vi "界面UI.vi"() -> ()   [LabVIEW 2016, in "德润DR803M超标留样.lvlib"]
uses:
  <vilib>/Utility/miscctls.llb/LVPointTypeDef.ctl
  <vilib>/Utility/config.llb/NI_LVConfig.lvlib
panel:
  in  "超标浓度配置":bool
  out "超标留样等待时间/s":dbl
  in  "流程停止":bool
  in  "流程启动":bool
  out "流程中":bool
  out "超标留样运行状态":T1(xcontrol)
  in  "外控留样设置":bool
  in  "外控留样读取":bool
  in  "串口重开":bool
  in  "读取选择":string(combo)
  in  "超标留样设置":bool
  in  "超标留样读取":bool
  in  "VISA resource name":refnum<visa-resource-name>="COM10" caption="VISA资源名称"
  in  "写入缓冲区":string
  in  "采样模式":enum16{"定时留样", "时间等比", "同步留样", "外控留样", "超标留样"}(ring)
  in  "采样启动":bool
  in  "切换停止":bool
  in  "切换运行":bool
  in  "时间校准":bool
  out "仪器状态":T1 {"仪器时间" format="%<%Y/%m/%d %H:%M:%S>T"; "门状态" items=["关闭", "打开"]; "采样模式" items=["定时留样"=1, "时间等比"=2, "同步留样"=3, "外控留样"=4, "超标留样"=5]; "工作进程" items=["停止中"=0, "启动延时"=1, "外置泵延时"=2, "管路润洗"=3, "管存"=4, "留样"=5, "出水管路排空"=6, "采水管路排空"=7, "待机"=13]; "工作状态" items=["停止", "运行", "系统初始化"]}
  out "读取缓冲区":string
  out "source":string
  out "通讯":bool
  # "德润超标留样803M"
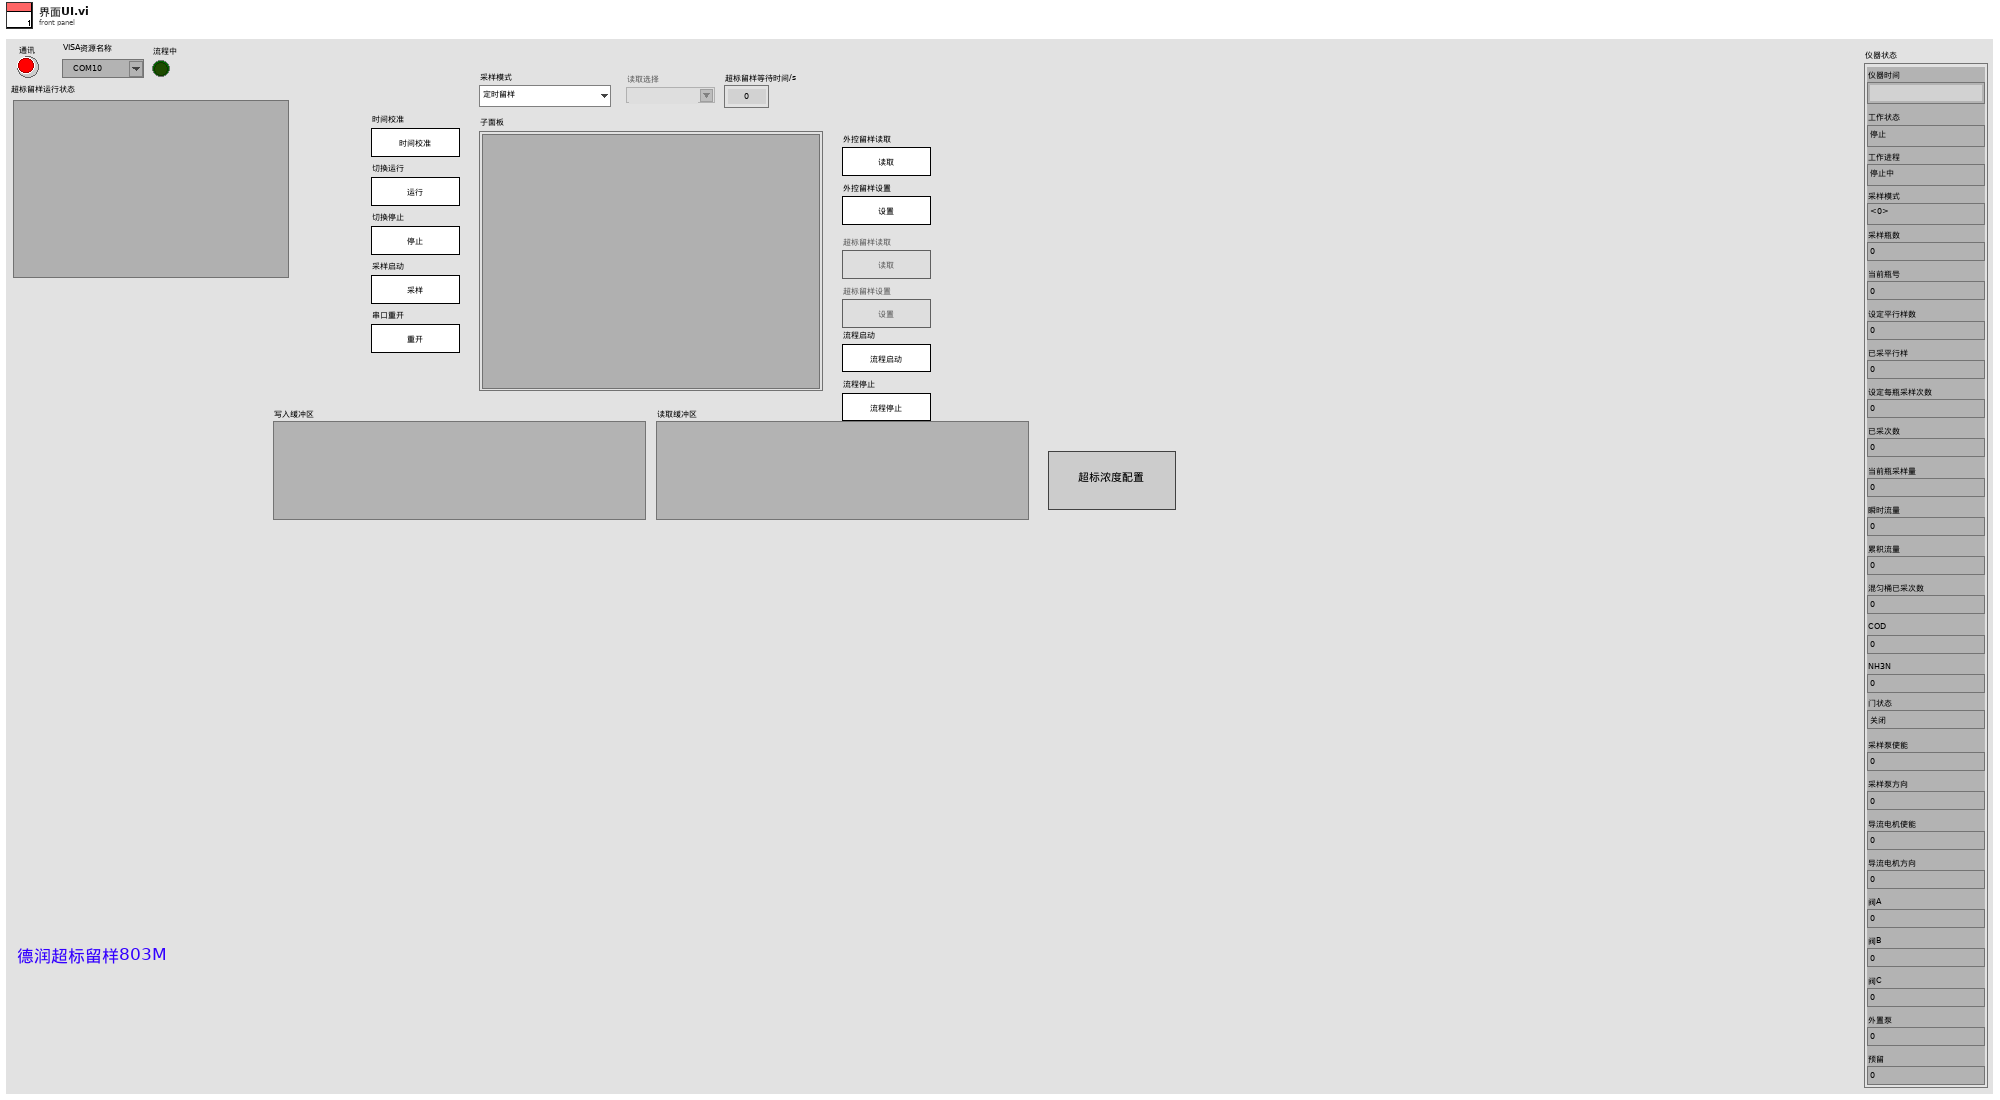
[diagram p1: front panel]
types:
  T1 = cluster{"仪器时间":timestamp, "工作状态":u16, "工作进程":u16, "采样模式":u16, "采样瓶数":dbl, "当前瓶号":dbl, "设定平行样数":dbl, "已采平行样":dbl, "设定每瓶采样次数":dbl, "已采次数":dbl, "当前瓶采样量":dbl, "瞬时流量":dbl, "累积流量":dbl, "混匀桶已采次数":dbl, "COD":dbl, "NH3N":dbl, "门状态":u16, "采样泵使能":dbl, "采样泵方向":dbl, "导流电机使能":dbl, "导流电机方向":dbl, "阀A":dbl, "阀B":dbl, "阀C":dbl, "外置泵":dbl, "预留":dbl}
  T2 = cluster{"STEP":enum16{"open", "read", "write", "close"}, "写入缓冲区":string}
  T3 = typedef "LVPointTypeDef.ctl" = cluster{"Horizontal":i16, "Vertical":i16}
  T4 = typedef "NI_LVConfig.lvlib/Config Data RefNum.ctl" = refnum<k1>
  T5 = enum32{"Bad", "Idle", "Run top level", "Running"}
  T6 = cluster{"当前瓶号：":dbl, "平行样：":dbl, "留样瓶数：":dbl, "每瓶次数：":dbl, "每次留样：":dbl}
  T7 = cluster{"当前瓶号：":dbl, "平行样：":dbl, "留样瓶数：":dbl, "每瓶次数：":dbl, "每次留样：":dbl, "时间间隔：":dbl, "COD联机：":u16, "氨氮联机：":u16, "4mA浓度：":dbl, "20mA浓度：":dbl, "超标浓度：":dbl, "4mA浓度：":dbl, "20mA浓度:":dbl, "超标浓度：":dbl}
  T8 = cluster{"[0]":dbl, "[1]":dbl, "[2]":dbl, "[3]":dbl, "[4]":dbl}
  T9 = cluster{"确定":bool, "氨氮超标浓度":dbl, "总磷超标浓度":dbl, "总氮超标浓度":dbl, "CODMn超标浓度":dbl, "CODCr超标浓度":dbl}
  T10 = enum8{"Enabled", "Disabled", "Disabled and Grayed Out"}
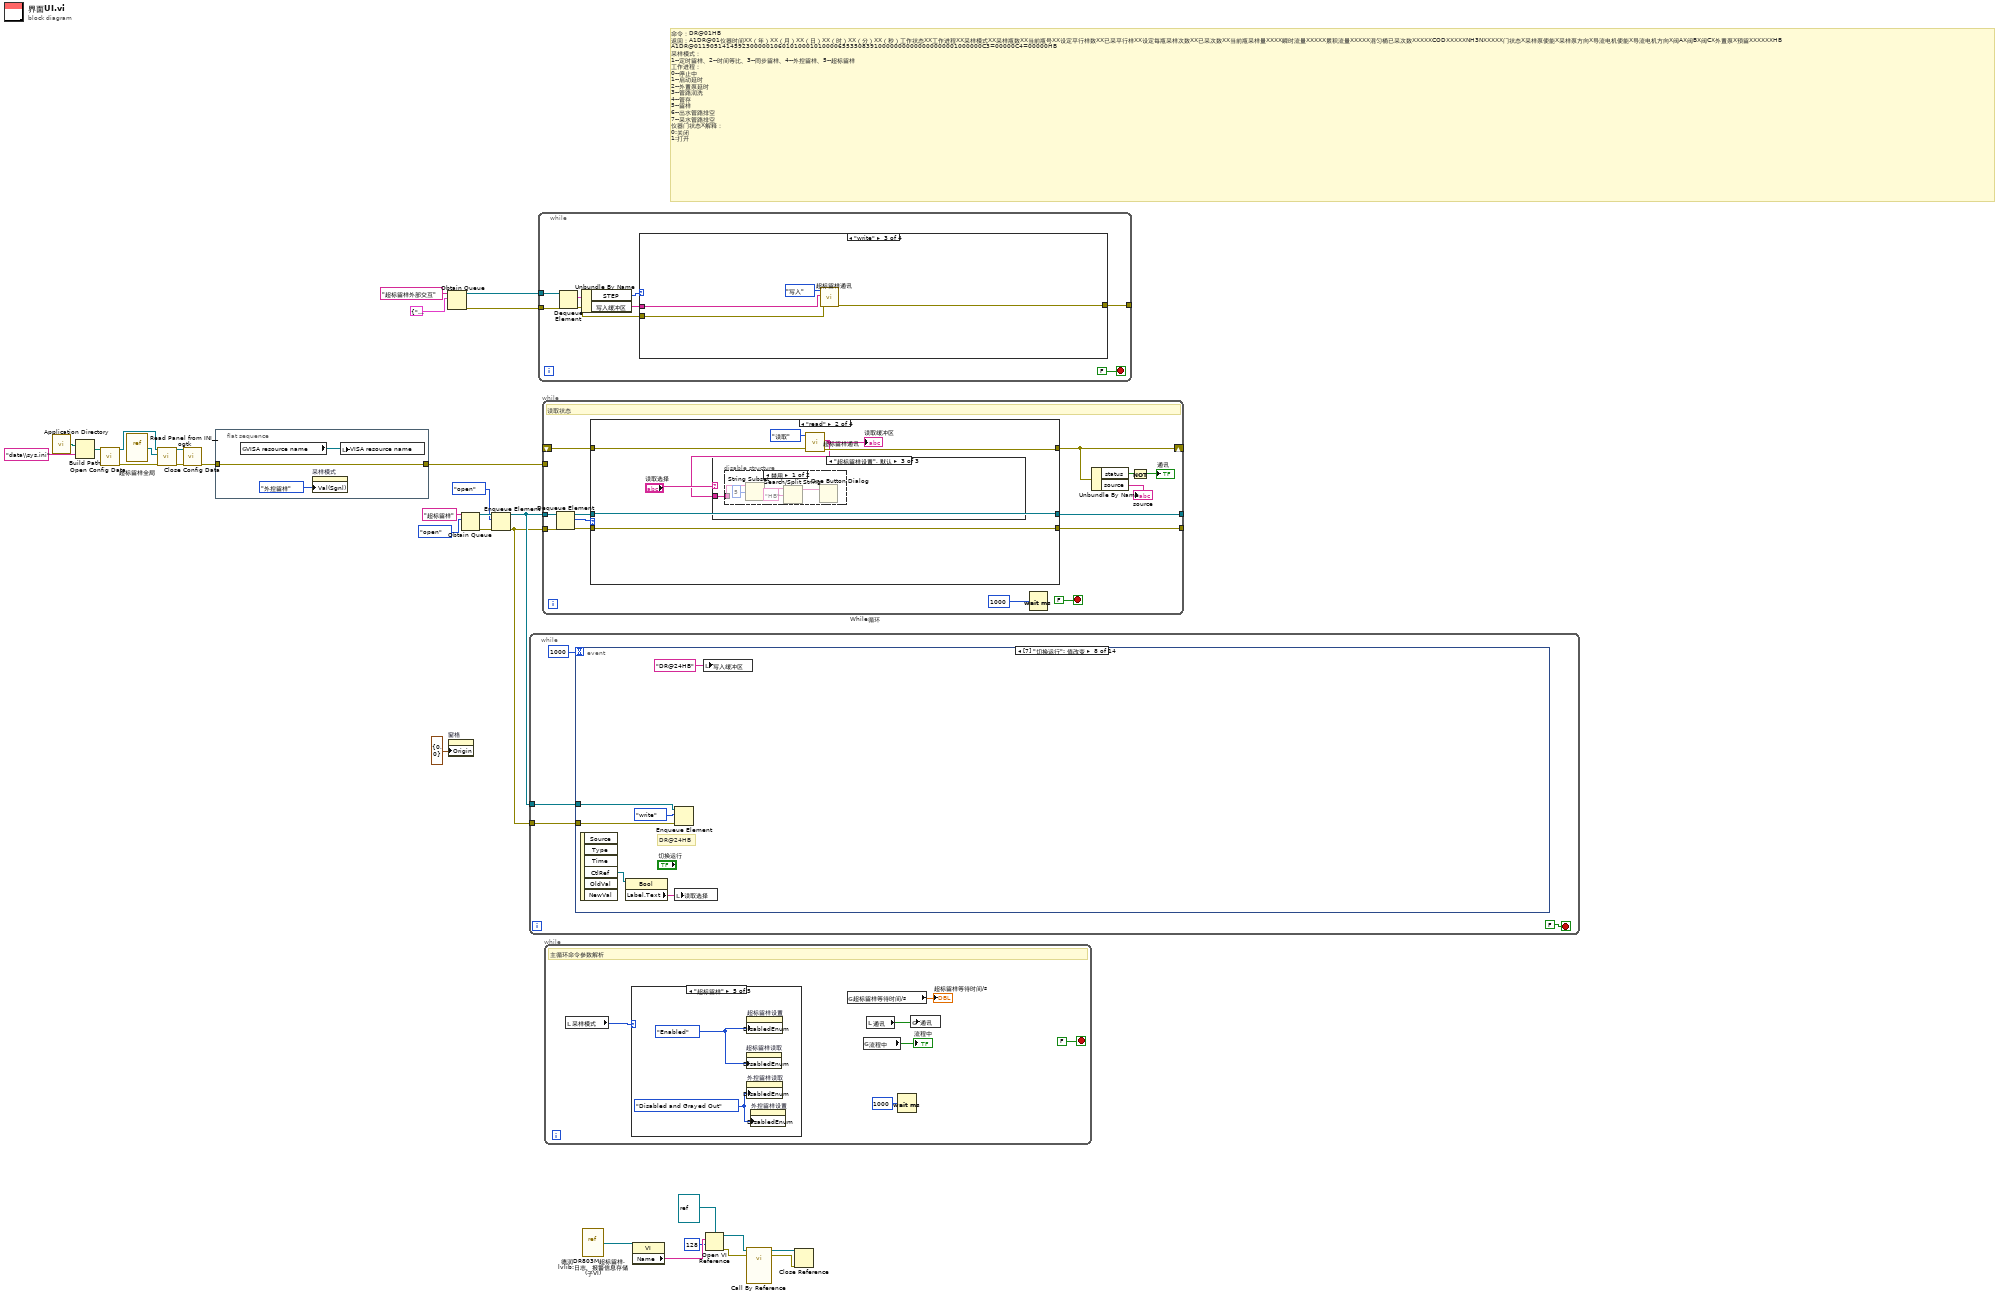
[diagram p0: block diagram]
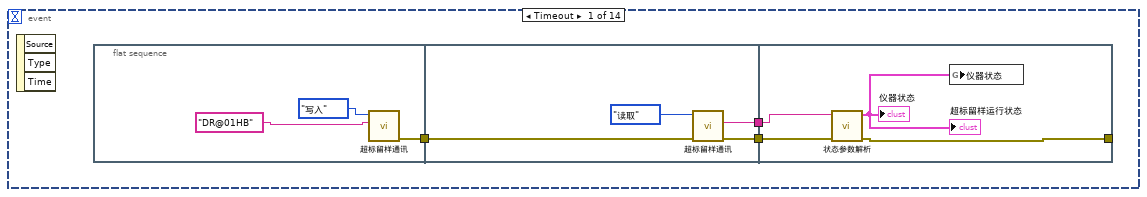
[diagram p5: hidden frame]
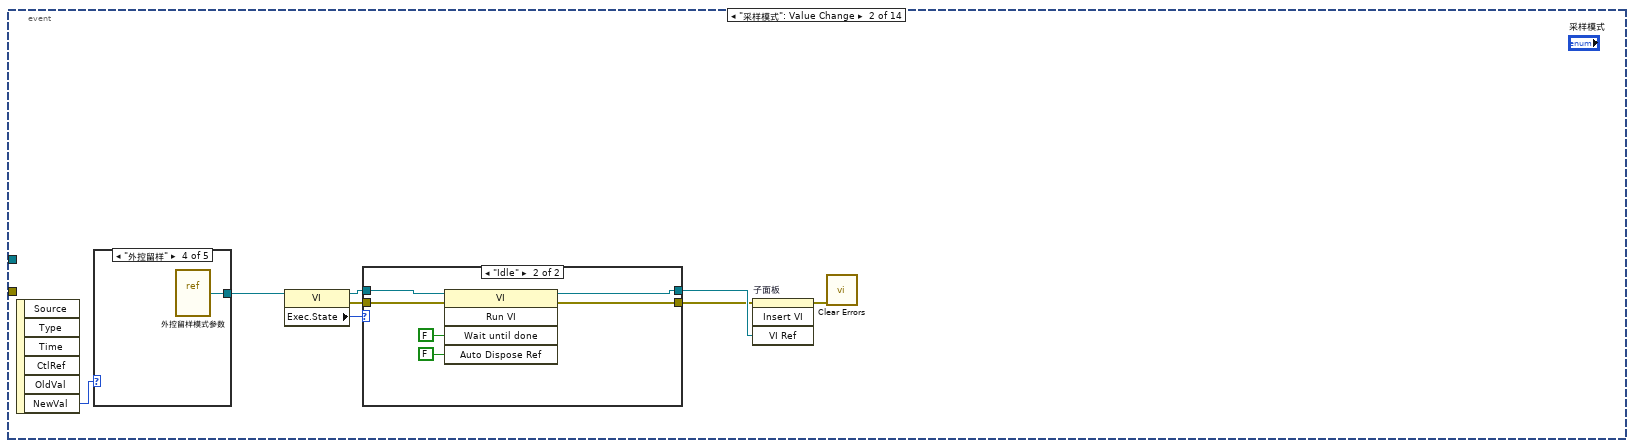
[diagram p6: hidden frame]
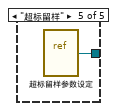
[diagram p11: hidden frame]
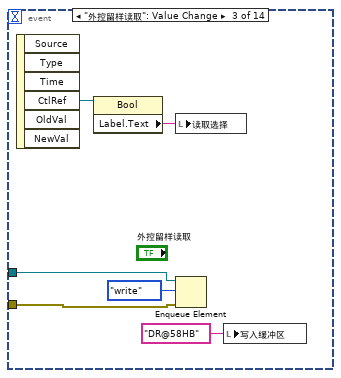
[diagram p12: hidden frame]
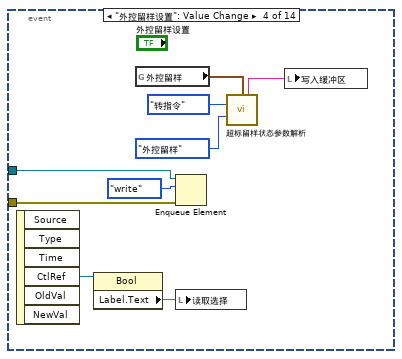
[diagram p13: hidden frame]
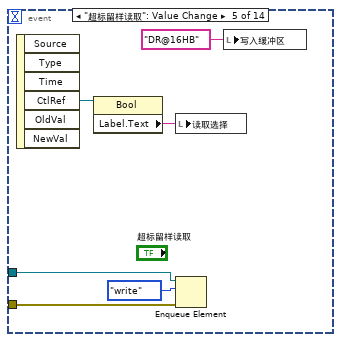
[diagram p14: hidden frame]
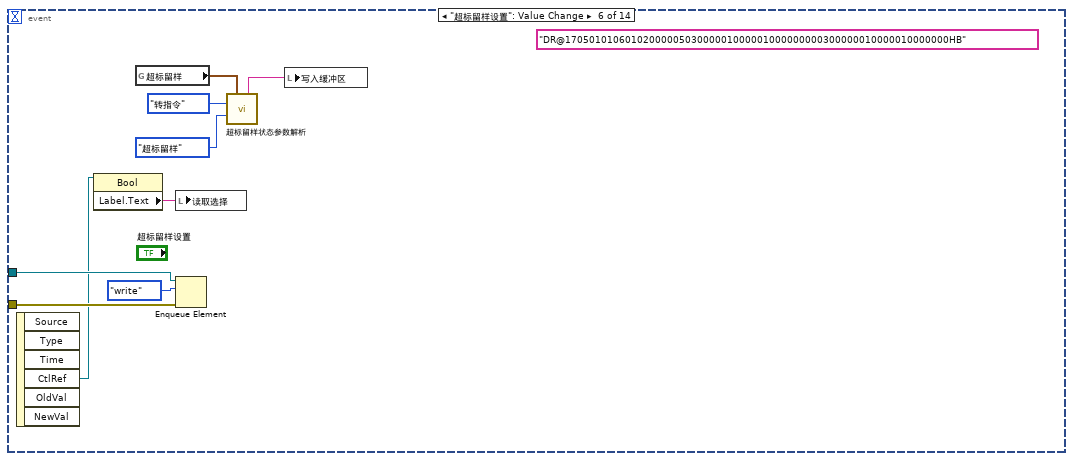
[diagram p15: hidden frame]
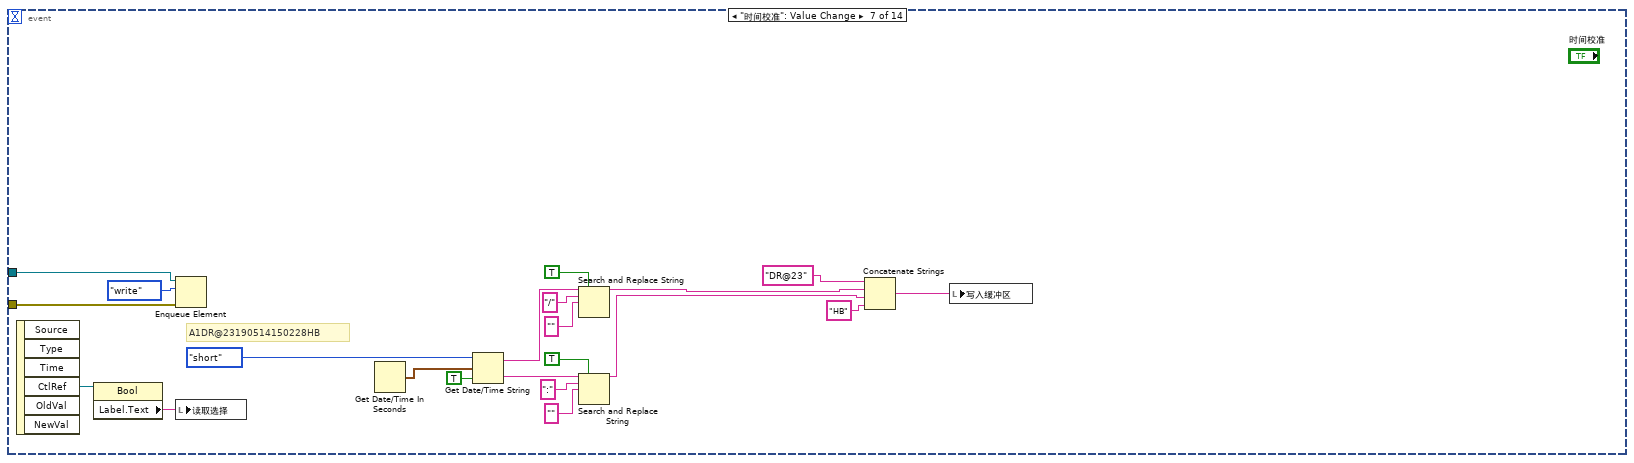
[diagram p16: hidden frame]
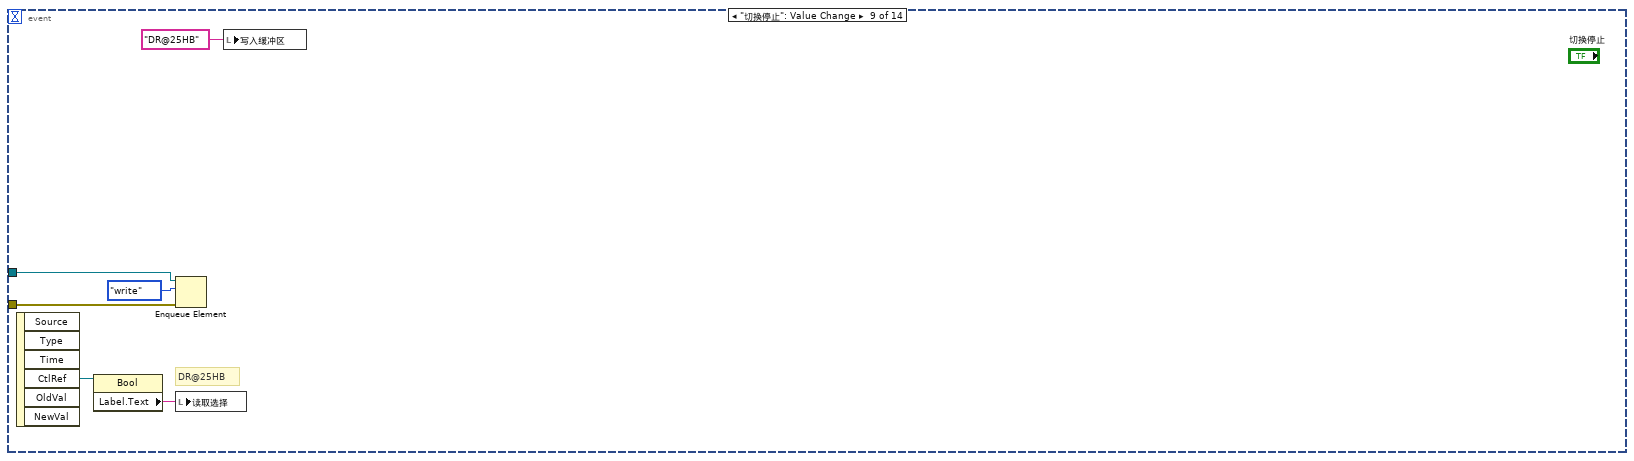
[diagram p17: hidden frame]
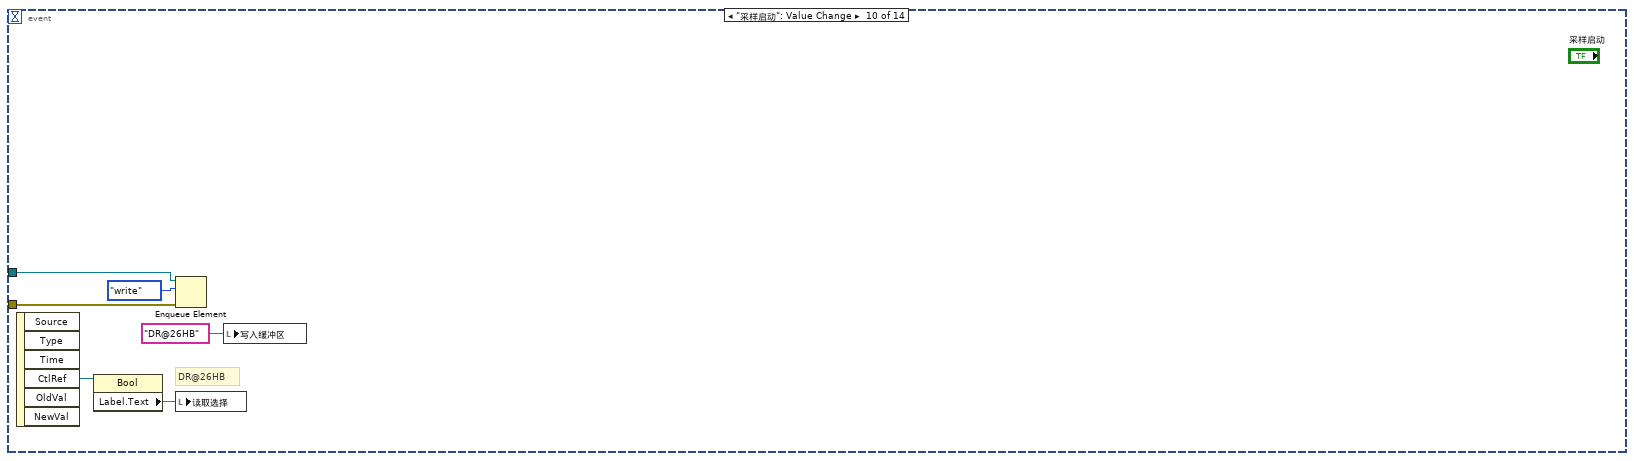
[diagram p18: hidden frame]
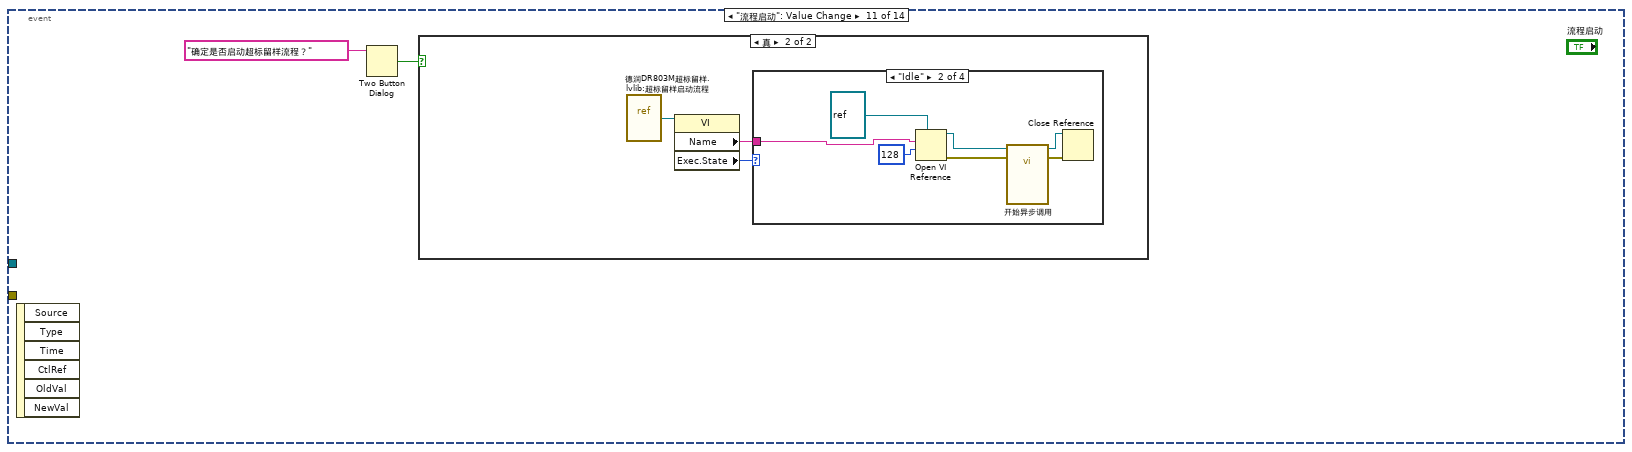
[diagram p19: hidden frame]
diagram:
  # "命令：DR@01HB\n返回：A1DR@01仪器时间XX（年）XX（月）XX（日）XX（时）XX（分）XX（秒）工作状态XX工作进程XX采样模式XX采样瓶数XX当前瓶号XX设定平行样数XX已采平行样XX设定每瓶采样次数XX已采次数XX当前瓶采样量XXXX瞬时流量XXXXX累积流量XXXXX混匀桶已采次数XXXXXCODXXXXXNH3NXXXXX门状态X采样泵使能X采样泵方向X导流电机使能X导流电机方向X阀AX阀BX阀CX外置泵X预留XXXXXXHB\nA1DR@011905141459230000010601010001010000655350839100000000000000000001000000C3=00000C4=00000HB\n采样模式：\n1--定时留样、2--时间等比、3--同步留样、4--外控留样、5--超标留样\n工作进程：\n0--停止中\n1--启动延时\n2--外置泵延时\n3--管路润洗\n4--管存\n5--留样\n6--出水管路排空\n7--采水管路排空\n仪器门状态X解释：\n0:关闭\n1:打开"
  n1 = call <vilib>:"Application Directory.vi"() -> ("Application Directory"=w22:path)
  n2 = Build Path(base path=w22, name or relative path="data\\sys.ini" ("名称或相对路径")) -> (appended path=w20:path)
  n3 = call <vilib>:"Open Config Data.vi"("configuration file path"=w20) -> ("error out"=w16:errorcluster, "refnum"=w19:T4)  [unwired: 8 in, 1 out]
  n4 = vi-ref "超标留样全局.vi"() -> (w18:refnum<vi>)
  n5 = call <userlib>:"Read Panel from INI__ogtk.vi"("error in (no error)"=w16, "VI ref"=w18, "refnum"=w19) -> ("error out"=w15:errorcluster, "refnum out"=w17:T4)  [unwired: 7 in]
  n6 = call <vilib>:"Close Config Data.vi"("error in (no error)"=w15, "refnum"=w17) -> ("error out"=w14:errorcluster)  [unwired: 8 in, 1 out]
  n7 = flat-sequence {
    tunnel: w14 -> [w33]
    tunnel: [w33] -> w13
    frame #0 {
      n8 = global read "超标留样全局.vi" "VISA resource name"() -> (w32:refnum<visa-resource-name>)
      n9 = property on="采样模式" class="Enum (严格)"("Val(Sgnl)"=enum16{"定时留样", "时间等比", "同步留样", "外控留样", "超标留样"}."外控留样" ("采样模式")) -> ()  [unwired: 2 in, 2 out]
      n10 = local write "VISA resource name"(w32) -> ()
    }
  }
  n11 = Obtain Queue(name (unnamed)="超标留样外部交互" ("名称（未命名）"), element data type=T2 {"STEP"=enum."write", "写入缓冲区"="ª\u0006\u0000\u0000P`\u00000»"}) -> (queue out=w11:refnum<queue>, error out=w10:errorcluster)  [unwired: 3 in, 1 out]
  n12 = property on="窗格" class="Pane"("Origin"=T3 {"Horizontal"=0, "Vertical"=0} ("原点")) -> ()  [unwired: 2 in, 2 out]
  n13 = Obtain Queue(name (unnamed)="超标留样" ("名称（未命名）"), element data type=enum16{"open", "read", "write", "close"}."open") -> (queue out=w28:refnum<queue>, error out=w27:errorcluster)  [unwired: 3 in, 1 out]
  n14 = Enqueue Element(queue=w28, element=enum16{"open", "read", "write", "close"}."open", error in (no error)=w27) -> (queue out=w25:refnum<queue>, error out=w24:errorcluster)  [unwired: 1 in, 1 out]
  n15 = while {
    tunnel: w25 -> [w36]
    tunnel: w24 -> [w35]
    stop <- FALSE stop-if-true
    n16 = event shown="[7] \"切换运行\": 值改变" {
      selector: _ -> [_ _ _ _ _ _ _ _ _ _ _ _ _ _]
      dyn-events: _ -> [_ _ _ _ _ _ _ _ _ _ _ _ _ _]
      timeout: 1000 -> [_ _ _ _ _ _ _ _ _ _ _ _ _ _]
      tunnel: w36 -> [_ _ w72 w83 w88 w98 w119 w124 w130 w136 _ w153 w168 _]
      tunnel: w35 -> [_ _ w73 w82 w87 w97 w118 w123 w129 w135 _ w152 w167 _]
      event Timeout {
        n17 = event-data() -> ()  [unwired: 1 in, 3 out]
        n18 = flat-sequence {
          tunnel: [w41] -> w40
          tunnel: w40 -> [w46]
          tunnel: [w45] -> w39
          tunnel: [w44] -> w38
          tunnel: w39 -> [w51]
          tunnel: w38 -> [w50]
          tunnel: [w49] -> _
          frame #0 {
            n19 = call "超标留样通讯.vi"("写入缓冲区"="DR@01HB", "功能输入"=enum16{"打开串口", "写入", "读取", "关闭串口"}."写入") -> ("error out"=w41:errorcluster)  [unwired: 7 in, 2 out]
          }
          frame #1 {
            n20 = call "超标留样通讯.vi"("error in (no error)"=w46, "功能输入"=enum16{"打开串口", "写入", "读取", "关闭串口"}."读取") -> ("error out"=w45:errorcluster, "读取缓冲区"=w44:string)  [unwired: 7 in, 1 out]
          }
          frame #2 {
            n21 = call "状态参数解析.vi"("error in (no error)"=w51, "字符串"=w50) -> ("error out"=w49:errorcluster, "簇"=w48:T1)  [unwired: 8 in]
            "仪器状态" <- w48
            "超标留样运行状态" <- w48
            n22 = global write "超标留样全局.vi" "仪器状态"(w48) -> ()
          }
        }
      }
      event "采样模式": Value Change {
        n23 = event-data() -> ("NewVal"=w59:enum16{"定时留样", "时间等比", "同步留样", "外控留样", "超标留样"})  [unwired: 1 in, 5 out]
        n24 = case shown="\"外控留样\"" w59 {
          tunnel: [_ _ _ w68 w69] -> w58
          frame "定时留样", Default {
          }
          frame "时间等比" {
          }
          frame "同步留样" {
          }
          frame "外控留样" {
            n25 = vi-ref "外控留样模式参数.vi"() -> (w68:refnum<vi>)
          }
          frame "超标留样" {
            n26 = vi-ref "超标留样参数设定.vi"() -> (w69:refnum<vi>)
          }
        }
        n27 = property class="VI"(reference=w58) -> (reference out=w56:refnum<vi>, error out=w54:errorcluster, "Exec.State"=w57:T5)  [unwired: 1 in]
        n28 = case shown="\"Idle\"" w57 {
          tunnel: w56 -> [w61 w67]
          tunnel: [w61 w64] -> w55
          tunnel: w54 -> [w60 w63]
          tunnel: [w60 w62] -> w53
          frame "Bad", Default {
          }
          frame "Idle" {
            n29 = invoke class="VI" method="Run VI"(reference=w67, error in=w63, "Wait until done"=FALSE ("结束前等待"), "Auto Dispose Ref"=FALSE ("自动销毁引用")) -> (reference out=w64:refnum<vi>, error out=w62:errorcluster)  [unwired: 1 in, 3 out]
          }
        }
        n30 = invoke on="子面板" class="SubPnl" method="Insert VI"(error in=w53, "VI Ref"=w55) -> (error out=w52:errorcluster)  [unwired: 2 in, 3 out]
        n31 = call <vilib>:"Clear Errors.vi"("error in (no error)"=w52) -> ()  [unwired: 5 in, 2 out]
      }
      event "外控留样读取": Value Change {
        n32 = event-data() -> ("CtlRef"=w71:refnum<vi>)  [unwired: 1 in, 5 out]
        n33 = property class="Bool"(reference=w71) -> ("Label.Text"=w70:string)  [unwired: 1 in, 2 out]
        n34 = local write "读取选择"(w70) -> ()
        n35 = Enqueue Element(queue=w72, element=enum16{"open", "read", "write", "close"}."write" ("元素"), error in (no error)=w73) -> ()  [unwired: 1 in, 3 out]
        n36 = local write "写入缓冲区"("DR@58HB") -> ()
      }
      event "外控留样设置": Value Change {
        n37 = event-data() -> ("CtlRef"=w77:refnum<vi>)  [unwired: 1 in, 5 out]
        n38 = property class="Bool"(reference=w77) -> ("Label.Text"=w76:string)  [unwired: 1 in, 2 out]
        n39 = global read "超标留样全局.vi" "外控留样"() -> (w78:T6)
        n40 = Enqueue Element(queue=w83, element=enum16{"open", "read", "write", "close"}."write" ("元素"), error in (no error)=w82) -> ()  [unwired: 1 in, 3 out]
        n41 = local write "读取选择"(w76) -> ()
        n42 = call "超标留样状态参数解析.vi"("外控留样"=w78, "解析/转指令"=enum16{"解析", "转指令"}."转指令", "模式选择"=enum16{"外控留样", "超标留样"}."外控留样") -> ("输出字符串"=w79:string)  [unwired: 11 in, 1 out]
        n43 = local write "写入缓冲区"(w79) -> ()
      }
      event "超标留样读取": Value Change {
        n44 = event-data() -> ("CtlRef"=w86:refnum<vi>)  [unwired: 1 in, 5 out]
        n45 = property class="Bool"(reference=w86) -> ("Label.Text"=w85:string)  [unwired: 1 in, 2 out]
        n46 = local write "读取选择"(w85) -> ()
        n47 = Enqueue Element(queue=w88, element=enum16{"open", "read", "write", "close"}."write" ("元素"), error in (no error)=w87) -> ()  [unwired: 1 in, 3 out]
        n48 = local write "写入缓冲区"("DR@16HB") -> ()
      }
      event "超标留样设置": Value Change {
        (unwired) "DR@1705010106010200000503000001000001000000000300000010000010000000HB"
        n49 = event-data() -> ("CtlRef"=w92:refnum<vi>)  [unwired: 1 in, 5 out]
        n50 = property class="Bool"(reference=w92) -> ("Label.Text"=w91:string)  [unwired: 1 in, 2 out]
        n51 = global read "超标留样全局.vi" "超标留样"() -> (w96:T7)
        n52 = local write "读取选择"(w91) -> ()
        n53 = Enqueue Element(queue=w98, element=enum16{"open", "read", "write", "close"}."write" ("元素"), error in (no error)=w97) -> ()  [unwired: 1 in, 3 out]
        n54 = call "超标留样状态参数解析.vi"("超标留样"=w96, "解析/转指令"=enum16{"解析", "转指令"}."转指令", "模式选择"=enum16{"外控留样", "超标留样"}."超标留样") -> ("输出字符串"=w93:string)  [unwired: 11 in, 1 out]
        n55 = local write "写入缓冲区"(w93) -> ()
      }
      event "时间校准": Value Change {
        # "A1DR@23190514150228HB"
        n56 = event-data() -> ("CtlRef"=w101:refnum<vi>)  [unwired: 1 in, 5 out]
        n57 = property class="Bool"(reference=w101) -> ("Label.Text"=w100:string)  [unwired: 1 in, 2 out]
        n58 = Enqueue Element(queue=w119, element=enum16{"open", "read", "write", "close"}."write" ("元素"), error in (no error)=w118) -> ()  [unwired: 1 in, 3 out]
        n59 = local write "读取选择"(w100) -> ()
        n60 = Get Date/Time In Seconds() -> (seconds since 1Jan1904=w114:timestamp)
        n61 = Get Date/Time String(date format (0)=enum16{"short", "long", "abbreviated"}."short" ("日期格式(0)"), seconds (now)=w114, want seconds? (F)=TRUE ("需要秒？(F)")) -> (date string=w113:string, time string=w106:string)
        n62 = Search and Replace String(replace all?=TRUE ("替换全部？(F)"), input string=w113, search string="/" ("搜索字符串"), replace string="" ("替换字符串(\"\")")) -> (result string=w105:string)  [unwired: 4 in, 3 out]
        n63 = Search and Replace String(replace all?=TRUE ("替换全部？(F)"), input string=w106, search string=":" ("搜索字符串"), replace string="" ("替换字符串(\"\")")) -> (result string=w104:string)  [unwired: 4 in, 3 out]
        n64 = Concatenate Strings("DR@23" ("写入缓冲区"), w105, w104, "HB" ("写入缓冲区")) -> (w102:string)
        n65 = local write "写入缓冲区"(w102) -> ()
      }
      event "切换运行": Value Change {
        # "DR@24HB"
        n66 = event-data() -> ("CtlRef"=w122:refnum<vi>)  [unwired: 1 in, 5 out]
        n67 = property class="Bool"(reference=w122) -> ("Label.Text"=w121:string)  [unwired: 1 in, 2 out]
        n68 = Enqueue Element(queue=w124, element=enum16{"open", "read", "write", "close"}."write" ("元素"), error in (no error)=w123) -> ()  [unwired: 1 in, 3 out]
        n69 = local write "读取选择"(w121) -> ()
        n70 = local write "写入缓冲区"("DR@24HB") -> ()
      }
      event "切换停止": Value Change {
        # "DR@25HB"
        n71 = event-data() -> ("CtlRef"=w128:refnum<vi>)  [unwired: 1 in, 5 out]
        n72 = property class="Bool"(reference=w128) -> ("Label.Text"=w127:string)  [unwired: 1 in, 2 out]
        n73 = Enqueue Element(queue=w130, element=enum16{"open", "read", "write", "close"}."write" ("元素"), error in (no error)=w129) -> ()  [unwired: 1 in, 3 out]
        n74 = local write "读取选择"(w127) -> ()
        n75 = local write "写入缓冲区"("DR@25HB" ("写入缓冲区")) -> ()
      }
      event "采样启动": Value Change {
        # "DR@26HB"
        n76 = event-data() -> ("CtlRef"=w134:refnum<vi>)  [unwired: 1 in, 5 out]
        n77 = property class="Bool"(reference=w134) -> ("Label.Text"=w133:string)  [unwired: 1 in, 2 out]
        n78 = Enqueue Element(queue=w136, element=enum16{"open", "read", "write", "close"}."write" ("元素"), error in (no error)=w135) -> ()  [unwired: 1 in, 3 out]
        n79 = local write "读取选择"(w133) -> ()
        n80 = local write "写入缓冲区"("DR@26HB") -> ()
      }
      event "流程启动": Value Change {
        n81 = event-data() -> ()  [unwired: 1 in, 6 out]
        n82 = Two Button Dialog(message="确定是否启动超标留样流程？" ("消息")) -> (T button?=w139:bool)  [unwired: 2 in]
        n83 = case shown="真" w139 {
          frame False {
          }
          frame True {
            n84 = vi-ref "德润DR803M超标留样.lvlib:超标留样启动流程.vi"() -> (w141:refnum<vi>)
            n85 = property class="VI"(reference=w141) -> ("Name"=w142:string, "Exec.State"=w143:T5)  [unwired: 1 in, 2 out]
            n86 = case shown="\"Idle\"" w143 {
              tunnel: w142 -> [_ w146 _ _]
              frame "Bad", Default {
              }
              frame "Idle" {
                n87 = Open VI Reference(type specifier VI Refnum (for type only)=refnum<vi> refnum ("类型说明符VI引用句柄（仅用于类型）"), vi path=w146, options=128 ("选项")) -> (vi reference=w150:refnum<vi>, error out=w145:errorcluster)  [unwired: 3 in]
                n88 = call-by-ref "开始异步调用"(reference=w150, error in=w145) -> (reference out=w149:refnum<vi>, error out=w144:errorcluster)  [unwired: 12 in]
                n89 = Close Reference(reference=w149, error in (no error)=w144) -> ()  [unwired: 1 out]
              }
              frame "Run top level" {
              }
              frame "Running" {
                n90 = One Button Dialog(message="流程已启动，无需重复启动！" ("消息")) -> ()  [unwired: 1 in, 1 out]
              }
            }
          }
        }
      }
      event "流程停止": Value Change {
        n91 = event-data() -> ()  [unwired: 1 in, 6 out]
        n92 = Two Button Dialog(message="确定是否停止超标留样流程并排空当前瓶？" ("消息")) -> (T button?=w154:bool)  [unwired: 2 in]
        n93 = case shown="真" w154 {
          tunnel: w153 -> [_ w158]
          tunnel: w152 -> [_ w157]
          frame False {
          }
          frame True {
            n94 = Enqueue Element(queue=w158, element=enum16{"open", "read", "write", "close"}."write" ("元素"), error in (no error)=w157) -> ()  [unwired: 1 in, 3 out]
            n95 = local write "写入缓冲区"("DR@25HB" ("写入缓冲区")) -> ()
            n96 = Obtain Notifier(name (unnamed)="超标留样流程" ("名称（未命名）"), notification data type=FALSE ("采样完成")) -> (notifier out=w164:refnum<notifier>, error out=w163:errorcluster)  [unwired: 2 in, 1 out]
            n97 = Send Notification(notification=TRUE ("通知"), notifier=w164, error in (no error)=w163) -> (notifier out=w161:refnum<notifier>, error out=w160:errorcluster)
            n98 = Release Notifier(notifier=w161, error in (no error)=w160) -> ()  [unwired: 1 in, 3 out]
          }
        }
      }
      event "串口重开": Value Change {
        n99 = event-data() -> ()  [unwired: 1 in, 6 out]
        n100 = flat-sequence {
          frame #0 {
            n101 = local read "VISA resource name"() -> (w170:refnum<visa-resource-name>)
            n102 = global write "超标留样全局.vi" "VISA resource name"(w170) -> ()
          }
          frame #1 {
            n103 = call <vilib>:"Application Directory.vi"() -> ("Application Directory"=w172:path)
            n104 = Build Path(base path=w172, name or relative path="data\\sys.ini" ("名称或相对路径")) -> (appended path=w173:path)
            n105 = call <vilib>:"Open Config Data.vi"("configuration file path"=w173) -> ("error out"=w177:errorcluster, "refnum"=w174:T4)  [unwired: 8 in, 1 out]
            n106 = vi-ref "超标留样全局.vi"() -> (w175:refnum<vi>)
            n107 = call <userlib>:"Write Panel to INI__ogtk.vi"("error in (no error)"=w177, "VI ref"=w175, "refnum"=w174) -> ("error out"=w178:errorcluster, "refnum out"=w176:T4)  [unwired: 7 in]
            n108 = call <vilib>:"Close Config Data.vi"("error in (no error)"=w178, "refnum"=w176) -> ("error out"=w183:errorcluster, "file path"=w184:path)  [unwired: 8 in]
            n109 = Open/Create/Replace File(file path (use dialog)=w184, error in=w183) -> (refnum out=w180:refnum<file>, error out=w179:errorcluster)  [unwired: 4 in, 1 out]
            n110 = Flush File(refnum=w180, error in=w179) -> (refnum out=w181:refnum<file>, error out=w182:errorcluster)
            n111 = Close File(refnum=w181, error in=w182) -> ()  [unwired: 2 out]
          }
        }
        n112 = Enqueue Element(queue=w168, element=enum16{"open", "read", "write", "close"}."close" ("元素"), error in (no error)=w167) -> ()  [unwired: 1 in, 3 out]
      }
      event "超标浓度配置": Value Change {
        n113 = event-data() -> ()  [unwired: 1 in, 6 out]
        n114 = global read "超标留样全局.vi" "CODMn超标浓度"() -> (w196:dbl)
        n115 = global read "超标留样全局.vi" "CODCr超标浓度"() -> (w197:dbl)
        n116 = global read "超标留样全局.vi" "氨氮超标浓度"() -> (w193:dbl)
        n117 = global read "超标留样全局.vi" "总磷超标浓度"() -> (w194:dbl)
        n118 = global read "超标留样全局.vi" "总氮超标浓度"() -> (w195:dbl)
        n119 = Build Array(w193, w194, w195, w196, w197) -> (w198:dbl[])
        n120 = Array To Cluster(array=w198) -> (cluster=w192:T8)
        n121 = call "超标浓度设置.vi"("输入"=w192) -> ("输出"=w191:T9)  [unwired: 10 in]
        n122 = Unbundle By Name(w191) -> ("确定"=w190:bool, "氨氮超标浓度"=w189:dbl, "总磷超标浓度"=w188:dbl, "总氮超标浓度"=w185:dbl, "CODMn超标浓度"=w186:dbl, "CODCr超标浓度"=w187:dbl)
        n123 = case shown="真" w190 {
          tunnel: w189 -> [_ w203]
          tunnel: w188 -> [_ w202]
          tunnel: w187 -> [_ w201]
          tunnel: w186 -> [_ w200]
          tunnel: w185 -> [_ w199]
          frame False {
          }
          frame True {
            n124 = flat-sequence {
              tunnel: w203 -> [w208]
              tunnel: w202 -> [w207]
              tunnel: w201 -> [w206]
              tunnel: w200 -> [w205]
              tunnel: w199 -> [w204]
              frame #0 {
                n125 = global write "超标留样全局.vi" "氨氮超标浓度"(w208) -> ()
                n126 = global write "超标留样全局.vi" "总磷超标浓度"(w207) -> ()
                n127 = global write "超标留样全局.vi" "总氮超标浓度"(w204) -> ()
                n128 = global write "超标留样全局.vi" "CODMn超标浓度"(w205) -> ()
                n129 = global write "超标留样全局.vi" "CODCr超标浓度"(w206) -> ()
              }
              frame #1 {
                n130 = call <vilib>:"Application Directory.vi"() -> ("Application Directory"=w210:path)
                n131 = Build Path(base path=w210, name or relative path="data\\sys.ini" ("名称或相对路径")) -> (appended path=w211:path)
                n132 = call <vilib>:"Open Config Data.vi"("configuration file path"=w211) -> ("error out"=w215:errorcluster, "refnum"=w212:T4)  [unwired: 8 in, 1 out]
                n133 = vi-ref "超标留样全局.vi"() -> (w213:refnum<vi>)
                n134 = call <userlib>:"Write Panel to INI__ogtk.vi"("error in (no error)"=w215, "VI ref"=w213, "refnum"=w212) -> ("error out"=w216:errorcluster, "refnum out"=w214:T4)  [unwired: 7 in]
                n135 = call <vilib>:"Close Config Data.vi"("error in (no error)"=w216, "refnum"=w214) -> ("error out"=w221:errorcluster, "file path"=w222:path)  [unwired: 8 in]
                n136 = Open/Create/Replace File(file path (use dialog)=w222, error in=w221) -> (refnum out=w218:refnum<file>, error out=w217:errorcluster)  [unwired: 4 in, 1 out]
                n137 = Flush File(refnum=w218, error in=w217) -> (refnum out=w219:refnum<file>, error out=w220:errorcluster)
                n138 = Close File(refnum=w219, error in=w220) -> ()  [unwired: 2 out]
              }
            }
          }
        }
      }
    }
  }
  n139 = while {
    tunnel: w11 -> [w230]
    tunnel: w10 -> [w229]
    tunnel: [w223] -> _
    stop <- FALSE stop-if-true
    n140 = Dequeue Element(queue=w230, error in (no error)=w229) -> (element=w227:T2, error out=w224:errorcluster)  [unwired: 1 in, 2 out]
    n141 = Unbundle By Name(w227) -> ("STEP"=w226:enum16{"open", "read", "write", "close"}, "写入缓冲区"=w225:string)
    n142 = case shown="\"write\"" w226 {
      tunnel: w225 -> [_ _ w234 _]
      tunnel: w224 -> [_ _ w232 _]
      tunnel: [_ _ w231 _] -> w223
      frame "open", Default {
      }
      frame "read" {
      }
      frame "write" {
        n143 = call "超标留样通讯.vi"("error in (no error)"=w232, "写入缓冲区"=w234, "功能输入"=enum16{"打开串口", "写入", "读取", "关闭串口"}."写入") -> ("error out"=w231:errorcluster)  [unwired: 6 in, 2 out]
      }
      frame "close" {
      }
    }
  }
  n144 = while "While循环" {
    tunnel: w25 -> [w246]
    tunnel: w24 -> [w245]
    tunnel: [w241] -> _
    tunnel: [w240] -> _
    shift-right: [w235] -> _
    shift-left: _ -> [w239]
    tunnel: w13 -> [_]
    stop <- FALSE stop-if-true
    # "读取状态"
    n145 = Dequeue Element(queue=w246, error in (no error)=w245) -> (queue out=w243:refnum<queue>, element=w244:enum16{"open", "read", "write", "close"}, error out=w242:errorcluster)  [unwired: 1 in, 1 out]
    n146 = case shown="\"read\"" w244 {
      tunnel: [w252 w259 w283 w295] -> w235
      tunnel: w243 -> [w251 w257 w288 w294]
      tunnel: w242 -> [w250 w256 w287 w293]
      tunnel: [w251 w257 w286 w291] -> w241
      tunnel: [w250 w256 w285 w290] -> w240
      tunnel: w239 -> [_ w260 w284 w297]
      frame "open", Default {
        (unwired) refnum<visa-resource-name> "COM2" ("VISA resource name")
        n147 = global write "超标留样全局.vi" "VISA resource name"("VISA resource name") -> ()
        n148 = call "超标留样通讯.vi"("VISA resource name"="VISA resource name", "功能输入"=enum16{"打开串口", "写入", "读取", "关闭串口"}."打开串口") -> ("error out"=w252:errorcluster)  [unwired: 7 in, 2 out]
      }
      frame "read" {
        n149 = call "超标留样通讯.vi"("error in (no error)"=w260, "功能输入"=enum16{"打开串口", "写入", "读取", "关闭串口"}."读取") -> ("error out"=w259:errorcluster, "读取缓冲区"=w254:string)  [unwired: 7 in, 1 out]
        "读取缓冲区" <- w254
        n150 = case shown="\"超标留样设置\", 默认" "读取选择" {
          tunnel: w254 -> [w261 w268 w275]
          frame "超标留样读取" {
            n151 = flat-sequence {
              tunnel: w261 -> [w264]
              frame #0 {
                n152 = call "超标留样状态参数解析.vi"("输入字符串"=w264, "解析/转指令"=enum16{"解析", "转指令"}."解析", "模式选择"=enum16{"外控留样", "超标留样"}."超标留样") -> ()  [unwired: 11 in, 2 out]
              }
              frame #1 {
                n153 = global write "超标留样全局.vi" "读取更新"(TRUE ("读取更新")) -> ()
              }
              frame #2 {
                n154 = Wait (ms)(milliseconds to wait=u32 500 ("等待时间（毫秒）")) -> ()  [unwired: 1 out]
              }
              frame #3 {
                n155 = global write "超标留样全局.vi" "读取更新"(FALSE ("读取更新")) -> ()
              }
            }
          }
          frame "外控留样读取" {
            n156 = flat-sequence {
              tunnel: w268 -> [w269]
              frame #0 {
                n157 = call "超标留样状态参数解析.vi"("输入字符串"=w269, "解析/转指令"=enum16{"解析", "转指令"}."解析", "模式选择"=enum16{"外控留样", "超标留样"}."外控留样") -> ()  [unwired: 11 in, 2 out]
              }
              frame #1 {
                n158 = global write "超标留样全局.vi" "外控留样读取更新"(TRUE ("读取更新")) -> ()
              }
              frame #2 {
                n159 = Wait (ms)(milliseconds to wait=u32 500 ("等待时间（毫秒）")) -> ()  [unwired: 1 out]
              }
              frame #3 {
                n160 = global write "超标留样全局.vi" "外控留样读取更新"(FALSE ("读取更新")) -> ()
              }
            }
          }
          frame "超标留样设置", Default {
            n161 = disable-structure shown="禁用" {
              disable-tunnel: w275 -> [w280 _]
              frame Disabled {
                n162 = String Subset(string=w280, offset (0)=5 ("偏移量(0)")) -> (substring=w278:string)  [unwired: 1 in]
                n163 = Search/Split String(string=w278, search string/char (-)="HB" ("搜索字符串/字符(-)")) -> (substring before match=w276:string)  [unwired: 1 in, 2 out]
                n164 = One Button Dialog(message=w276) -> ()  [unwired: 1 in, 1 out]
              }
              frame Enabled {
              }
            }
          }
        }
      }
      frame "write" {
        n165 = call "超标留样通讯.vi"("error in (no error)"=w284, "写入缓冲区"="写入缓冲区", "功能输入"=enum16{"打开串口", "写入", "读取", "关闭串口"}."写入") -> ("error out"=w283:errorcluster)  [unwired: 6 in, 2 out]
        n166 = Enqueue Element(queue=w288, element=enum16{"open", "read", "write", "close"}."read" ("元素"), error in (no error)=w287) -> (queue out=w286:refnum<queue>, error out=w285:errorcluster)  [unwired: 1 in, 1 out]
      }
      frame "close" {
        n167 = call "超标留样通讯.vi"("error in (no error)"=w297, "功能输入"=enum16{"打开串口", "写入", "读取", "关闭串口"}."关闭串口") -> ("error out"=w295:errorcluster)  [unwired: 7 in, 2 out]
        n168 = Enqueue Element(queue=w294, element=enum16{"open", "read", "write", "close"}."open" ("元素"), error in (no error)=w293) -> (queue out=w291:refnum<queue>, error out=w290:errorcluster)  [unwired: 1 in, 1 out]
      }
    }
    n169 = Wait (ms)(milliseconds to wait=u32 1000 ("等待时间（毫秒）")) -> ()  [unwired: 1 out]
    n170 = Unbundle By Name(w235) -> ("status"=w236:bool, "source"=→"source":string)
    n171 = Not(x=w236) -> (.not. x?=→"通讯":bool)
  }
  n172 = while {
    stop <- FALSE stop-if-true
    # "主循环命令参数解析"
    n173 = local read "采样模式"() -> (w301:enum16{"定时留样", "时间等比", "同步留样", "外控留样", "超标留样"})
    n174 = case shown="\"超标留样\"" w301 {
      frame "定时留样", Default {
        w304 = T10."Disabled and Grayed Out" ("禁用")
        n175 = property on="超标留样读取" class="Bool"("DisabledEnum"=w304) -> ()  [unwired: 2 in, 2 out]
        n176 = property on="超标留样设置" class="Bool"("DisabledEnum"=w304) -> ()  [unwired: 2 in, 2 out]
        n177 = property on="外控留样读取" class="Bool"("DisabledEnum"=w304) -> ()  [unwired: 2 in, 2 out]
        n178 = property on="外控留样设置" class="Bool"("DisabledEnum"=w304) -> ()  [unwired: 2 in, 2 out]
      }
      frame "时间等比" {
      }
      frame "同步留样" {
      }
      frame "外控留样" {
        w305 = T10."Enabled" ("禁用")
        w306 = T10."Disabled and Grayed Out" ("禁用")
        n179 = property on="超标留样读取" class="Bool"("DisabledEnum"=w306) -> ()  [unwired: 2 in, 2 out]
        n180 = property on="超标留样设置" class="Bool"("DisabledEnum"=w306) -> ()  [unwired: 2 in, 2 out]
        n181 = property on="外控留样读取" class="Bool"("DisabledEnum"=w305) -> ()  [unwired: 2 in, 2 out]
        n182 = property on="外控留样设置" class="Bool"("DisabledEnum"=w305) -> ()  [unwired: 2 in, 2 out]
      }
      frame "超标留样" {
        w307 = T10."Enabled" ("禁用")
        w308 = T10."Disabled and Grayed Out" ("禁用")
        n183 = property on="超标留样读取" class="Bool"("DisabledEnum"=w307) -> ()  [unwired: 2 in, 2 out]
        n184 = property on="超标留样设置" class="Bool"("DisabledEnum"=w307) -> ()  [unwired: 2 in, 2 out]
        n185 = property on="外控留样读取" class="Bool"("DisabledEnum"=w308) -> ()  [unwired: 2 in, 2 out]
        n186 = property on="外控留样设置" class="Bool"("DisabledEnum"=w308) -> ()  [unwired: 2 in, 2 out]
      }
    }
    n187 = global read "超标留样全局.vi" "超标留样等待时间/s"() -> (→"超标留样等待时间/s":dbl)
    n188 = global read "超标留样全局.vi" "流程中"() -> (→"流程中":bool)
    n189 = local read "通讯"() -> (w300:bool)
    n190 = Wait (ms)(milliseconds to wait=u32 1000 ("等待时间（毫秒）")) -> ()  [unwired: 1 out]
    n191 = global write "超标留样全局.vi" "通讯"(w300) -> ()
  }
  n192 = vi-ref "德润DR803M超标留样.lvlib:日志、报警信息存储 (子VI).vi"() -> (w8:refnum<vi>)
  n193 = property class="VI"(reference=w8) -> ("Name"=w7:string)  [unwired: 1 in, 2 out]
  n194 = Open VI Reference(type specifier VI Refnum (for type only)=refnum<vi> refnum ("类型说明符VI引用句柄（仅用于类型）"), vi path=w7, options=128 ("选项")) -> (vi reference=w5:refnum<vi>, error out=w3:errorcluster)  [unwired: 3 in]
  n195 = call-by-ref "?"(reference=w5, error in=w3) -> (reference out=w2:refnum<vi>, error out=w1:errorcluster)  [unwired: 12 in]
  n196 = Close Reference(reference=w2, error in (no error)=w1) -> ()  [unwired: 1 out]
